vi "FEA_Model_Pinned_BC.vi"(10 "Pin Location":i32, 11 "FEA_Model in":refnum<class "FEA_Model.lvclass">) -> (2 "K Matrix":dbl[][](array[numeric]), 3 "M Matrix":dbl[][](array[numeric]))   [LabVIEW 2021, in "FEA_Model.lvclass"]
uses:
  FEA_Model.lvclass
  FEA_Model.lvclass/FEA_Model.ctl
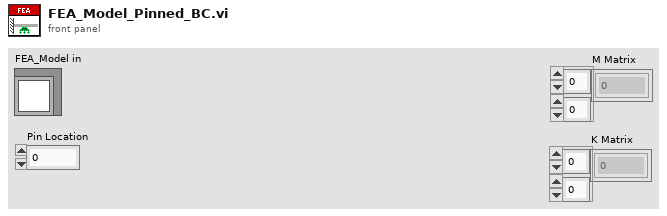
[diagram p1: front panel]
types:
  T1 = enum16{"Particles to Nodes", "Particle to Node", "Nodes to Particles", "Node to Particle"}
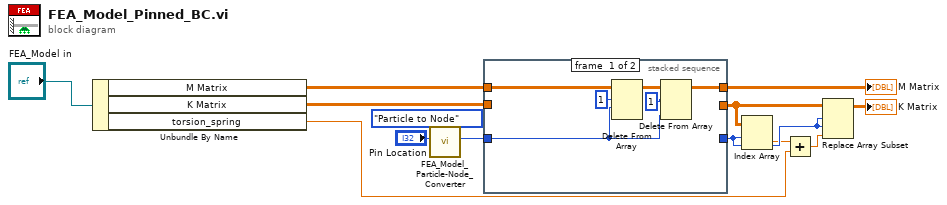
[diagram p0: block diagram]
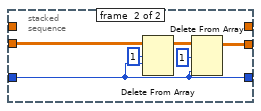
[diagram p2: hidden frame]
diagram:
  n1 = Unbundle By Name("FEA_Model in") -> ("M Matrix"=w12:dbl[][], "K Matrix"=w11:dbl[][], "torsion_spring"=w8:dbl)
  n2 = call "FEA_Model_Particle-Node_Converter.vi"("mode"=T1."Particle to Node", "Particle"="Pin Location") -> ("Node"=w1:i32)  [unwired: 6 in, 3 out]
  n3 = stacked-sequence {
    tunnel: [w19 _] -> w5
    tunnel: w12 -> [w16 _]
    tunnel: w1 -> [w14 w20]
    tunnel: w11 -> [_ w22]
    tunnel: [_ w21] -> w10
    tunnel: [_ w20] -> w9
    frame #0 {
      n4 = Delete From Array(array=w16, length=1, index (row)=w14) -> (array with subset deleted=w18:dbl[][])  [unwired: 1 in, 1 out]
      n5 = Delete From Array(array=w18, length=1, index (col)=w14) -> (array with subset deleted=w19:dbl[][])  [unwired: 1 in, 1 out]
    }
    frame #1 {
      n6 = Delete From Array(array=w22, length=1, index (row)=w20) -> (array with subset deleted=w25:dbl[][])  [unwired: 1 in, 1 out]
      n7 = Delete From Array(array=w25, length=1, index (col)=w20) -> (array with subset deleted=w21:dbl[][])  [unwired: 1 in, 1 out]
    }
  }
  "M Matrix" <- w5
  n8 = Index Array(array=w10, index (row)=w9, index (col)=w9) -> (element=w7:dbl)
  n9 = Add(x=w7, y=w8) -> (x+y=w6:dbl)
  n10 = Replace Array Subset(array=w10, new element=w6, index (row)=w9, index (col)=w9) -> (→"K Matrix":dbl[][])
